vi "Write Serial Port.vi"(8 "error in (no error)":errorcluster, 10 "Serial Port":refnum<visa-resource-name>, 11 "NXP LPCXpresso54608 in":refnum<class "NXP LPCXpresso54608.lvclass">) -> (0 "error out":errorcluster, 3 "NXP LPCXpresso54608 out":refnum<class "NXP LPCXpresso54608.lvclass">)   [LabVIEW 2020, in "NXP LPCXpresso54608.lvclass"]
uses:
  NXP LPCXpresso54608.lvclass
  NXP LPCXpresso54608.lvclass/NXP LPCXpresso54608.ctl
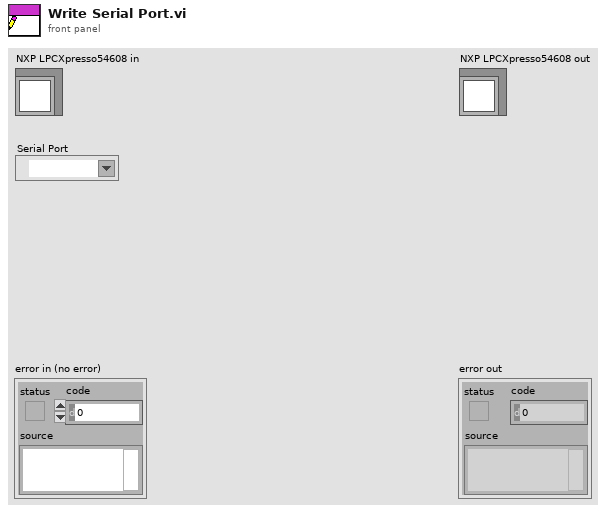
[diagram p1: front panel]
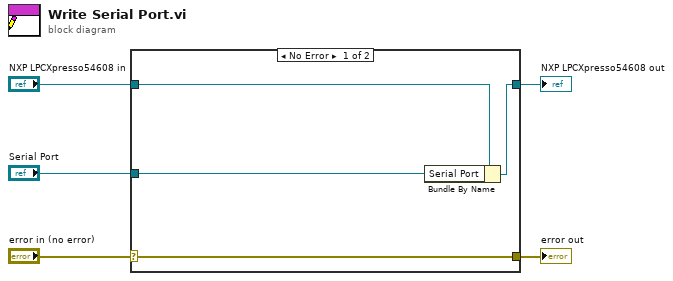
[diagram p0: block diagram]
diagram:
  n1 = case shown="No Error" "error in (no error)" {
    selector: "error in (no error)" -> [w9 w10]
    tunnel: [w9 w10] -> w4
    tunnel: [w7 w11] -> w2
    tunnel: "NXP LPCXpresso54608 in" -> [w8 w11]
    tunnel: "Serial Port" -> [w6 _]
    frame No Error {
      n2 = Bundle By Name(cluster=w8, "Serial Port"=w6) -> (w7:refnum<class "NXP LPCXpresso54608.lvclass">)
    }
    frame Error {
    }
  }
  "error out" <- w4
  "NXP LPCXpresso54608 out" <- w2
